vi "GetTime.vi"(8 "error in":errorcluster) -> (0 "error out":errorcluster, 2 "TimeCluster":T2, 3 "Local Data/Time[String]":T1)   [LabVIEW 2021, in "Time.lvlib"]
uses:
  Time.lvlib
  TypeDef/TimeCluster.ctl
  TypeDef/Local_DateTime_String.ctl
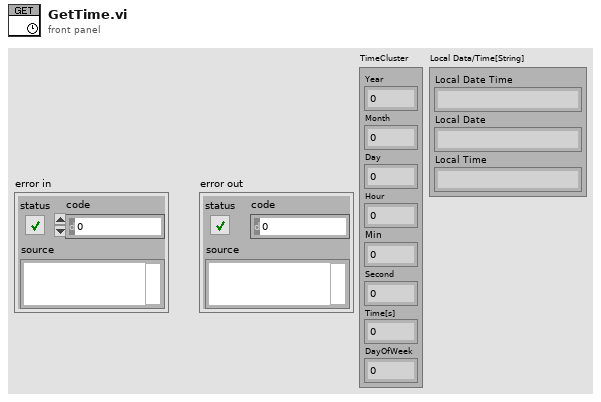
[diagram p1: front panel]
types:
  T1 = typedef "Time.lvlib/Local_DateTime_String.ctl" = cluster{"Local Date Time":string, "Local Date":string, "Local Time":string}
  T2 = typedef "Time.lvlib/TimeCluster.ctl" = cluster{"Year":i32, "Month":i32, "Day":i32, "Hour":i32, "Min":i32, "Second":i32, "Time[s]":i32, "DayOfWeek":i32}
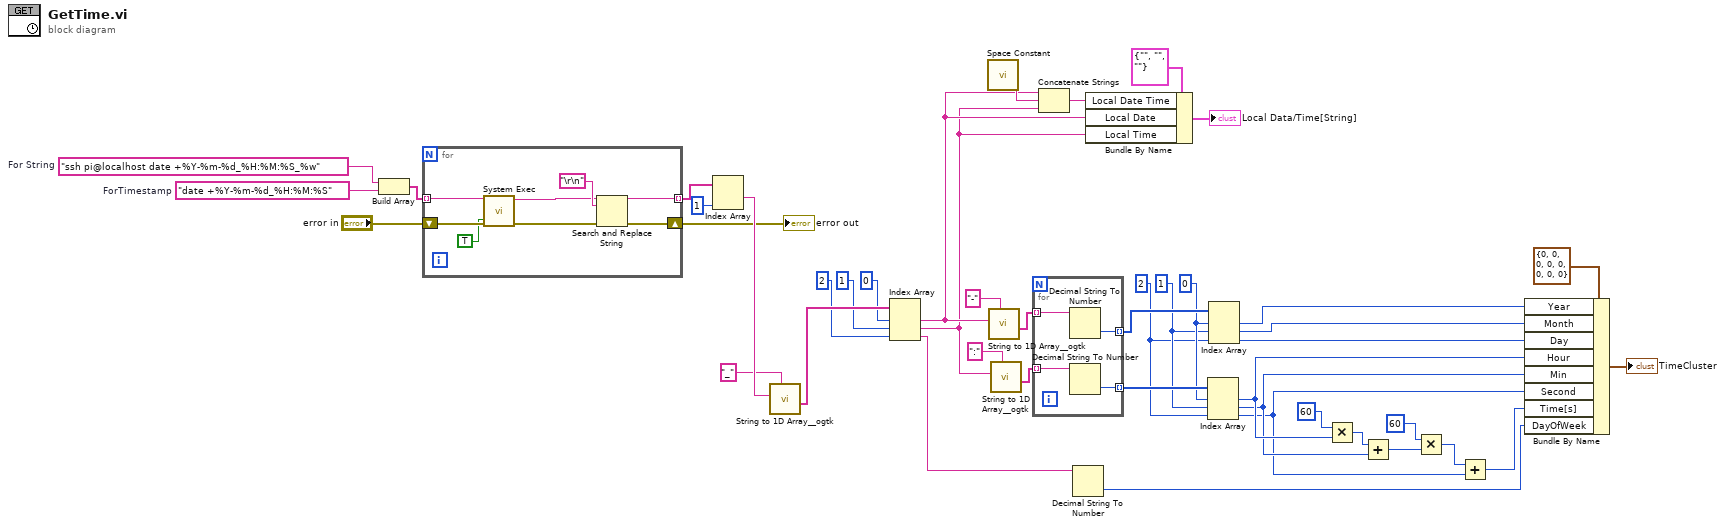
[diagram p0: block diagram]
diagram:
  w27 = 2 ("index")
  w28 = 1 ("index")
  w29 = 0 ("index")
  w41 = "ssh pi@localhost date +%Y-%m-%d_%H:%M:%S_%w"  # For String
  w43 = "date +%Y-%m-%d_%H:%M:%S"  # ForTimestamp
  n1 = Build Array(w41, w43) -> (w42:string[])
  n2 = for {
    shift-right: [w45] -> w1
    shift-left: "error in" -> [w52]
    tunnel: w42 -> [w51] mode=indexing
    tunnel: [w49] -> w40 mode=indexing
    n3 = call <vilib>:"System Exec.vi"("run minimized? (F)"=TRUE, "error in (no error)"=w52, "command line"=w51) -> ("error out"=w46:errorcluster, "standard output"=w47:string)  [unwired: 5 in, 2 out]
    n4 = Search and Replace String(input string=w47, search string="\r\n", error in=w46) -> (result string=w49:string, error out=w45:errorcluster)  [unwired: 5 in, 2 out]
  }
  "error out" <- w1
  n5 = Index Array(array=w40, index #2=1 ("index")) -> (element #1=w13:string)  [unwired: 1 in, 1 out]
  n6 = call <userlib>:"String to 1D Array__ogtk.vi"("delimiter (Tab)"="_" ("search string"), "string"=w13) -> ("Array of Strings"=w11:string[])  [unwired: 9 in]
  n7 = Index Array(array=w11, index #1=0 ("index"), index #2=1 ("index"), index #3=2 ("index")) -> (element #1=w5:string, element #2=w4:string, element #3=w3:string)
  n8 = call <vilib>:"Space Constant.vi"() -> ("String"=w6:string)
  n9 = call <userlib>:"String to 1D Array__ogtk.vi"("delimiter (Tab)"="-", "string"=w5) -> ("Array of Strings"=w36:string[])  [unwired: 9 in]
  n10 = call <userlib>:"String to 1D Array__ogtk.vi"("delimiter (Tab)"=":", "string"=w4) -> ("Array of Strings"=w35:string[])  [unwired: 9 in]
  n11 = for {
    tunnel: w36 -> [w56] mode=indexing
    tunnel: w35 -> [w55] mode=indexing
    tunnel: [w54] -> w34 mode=indexing
    tunnel: [w53] -> w33 mode=indexing
    n12 = Decimal String To Number(string=w56) -> (number=w54:i32)  [unwired: 2 in, 1 out]
    n13 = Decimal String To Number(string=w55) -> (number=w53:i32)  [unwired: 2 in, 1 out]
  }
  n14 = Concatenate Strings(w5, w6, w4) -> (w7:string)
  n15 = Decimal String To Number(string=w3) -> (number=w2:i32)  [unwired: 2 in, 1 out]
  n16 = Bundle By Name(cluster=T1 {"Local Date Time"="", "Local Date"="", "Local Time"=""} ("Local Data/Time[String]"), "Local Date Time"=w7, "Local Date"=w5, "Local Time"=w4) -> (→"Local Data/Time[String]":T1)
  n17 = Index Array(array=w33, index #1=w29, index #2=w28, index #3=w27) -> (element #1=w21:i32, element #2=w20:i32, element #3=w19:i32)
  n18 = Index Array(array=w34, index #1=w29, index #2=w28, index #3=w27) -> (element #1=w32:i32, element #2=w31:i32, element #3=w30:i32)
  n19 = Multiply(x=60, y=w21) -> (x*y=w25:i32)
  n20 = Add(x=w25, y=w20) -> (x+y=w23:i32)
  n21 = Multiply(x=60, y=w23) -> (x*y=w22:i32)
  n22 = Add(x=w22, y=w19) -> (x+y=w17:i32)
  n23 = Bundle By Name(cluster=T2 {"Year"=0, "Month"=0, "Day"=0, "Hour"=0, "Min"=0, "Second"=0, "Time[s]"=0, "DayOfWeek"=0} ("TimeCluster"), "Year"=w32, "Month"=w31, "Day"=w30, "Hour"=w21, "Min"=w20, "Second"=w19, "Time[s]"=w17, "DayOfWeek"=w2) -> (→"TimeCluster":T2)
